vi "GenerateChunks.vi"(9 "Empty Chunk":cluster{cluster{"Last Update":u32, bool}[][][]}, 10 "Point chunk":i32[](array[numeric]), 11 "Map Data in":T1(array[cluster])) -> (3 "Map Data out":T1(array[cluster]))   [LabVIEW 2014]
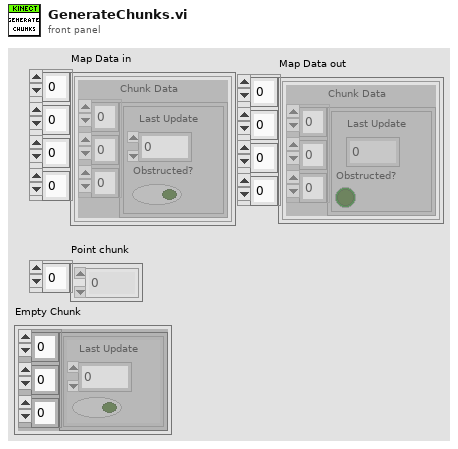
[diagram p1: front panel]
types:
  T1 = cluster{"Chunk Data":cluster{"Last Update":u32, "Obstructed?":bool}[][][]}[][][][]
  T2 = cluster{cluster{"Last Update":u32, bool}[][][]}[][][]
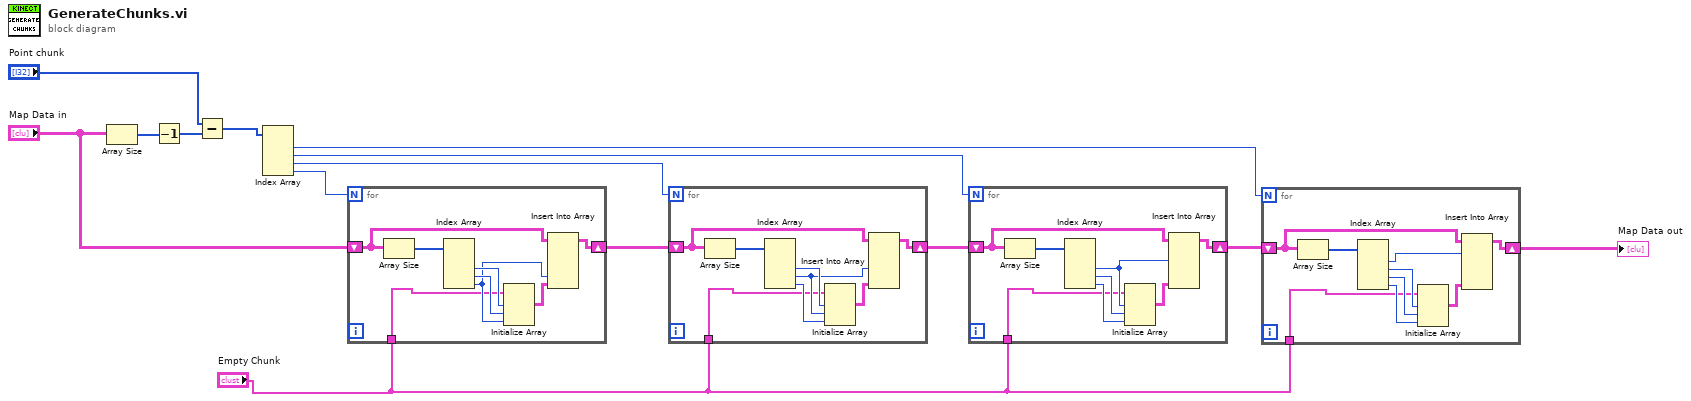
[diagram p0: block diagram]
diagram:
  n1 = Array Size(array="Map Data in") -> (size(s)=w14:i32[])
  n2 = Decrement(x=w14) -> (x-1=w13:i32[])
  n3 = Subtract(x="Point chunk", y=w13) -> (x-y=w4:i32[])
  n4 = Index Array(array=w4) -> (element #1=w11:i32, element #2=w9:i32, element #3=w7:i32, element #4=w6:i32)  [unwired: 4 in]
  n5 = for {
    N: w6 -> [_]
    shift-right: [w22] -> w5
    shift-left: "Map Data in" -> [w19]
    tunnel: "Empty Chunk" -> [w15]
    n6 = Array Size(array=w19) -> (size(s)=w21:i32[])
    n7 = Index Array(array=w21) -> (element #2=w17:i32, element #3=w18:i32, element #4=w16:i32)  [unwired: 4 in, 1 out]
    n8 = Initialize Array(w15, w17, w18, w16) -> (w20:T2)
    n9 = Insert Into Array(array=w19, index (dim 3)=w16, new element=w20) -> (w22:T1)  [unwired: 3 in]
  }
  n10 = for {
    N: w7 -> [_]
    shift-right: [w30] -> w8
    shift-left: w5 -> [w27]
    tunnel: "Empty Chunk" -> [w23]
    n11 = Array Size(array=w27) -> (size(s)=w29:i32[])
    n12 = Index Array(array=w29) -> (element #2=w25:i32, element #3=w24:i32, element #4=w26:i32)  [unwired: 4 in, 1 out]
    n13 = Initialize Array(w23, w25, w24, w26) -> (w28:T2)
    n14 = Insert Into Array(array=w27, index (dim 2)=w24, new element=w28) -> (w30:T1)  [unwired: 3 in]
  }
  n15 = for {
    N: w9 -> [_]
    shift-right: [w38] -> w10
    shift-left: w8 -> [w35]
    tunnel: "Empty Chunk" -> [w31]
    n16 = Array Size(array=w35) -> (size(s)=w37:i32[])
    n17 = Index Array(array=w37) -> (element #2=w32:i32, element #3=w34:i32, element #4=w33:i32)  [unwired: 4 in, 1 out]
    n18 = Initialize Array(w31, w32, w34, w33) -> (w36:T2)
    n19 = Insert Into Array(array=w35, index (dim 1)=w32, new element=w36) -> (w38:T1)  [unwired: 3 in]
  }
  n20 = for {
    N: w11 -> [_]
    shift-right: [w47] -> w1
    shift-left: w10 -> [w44]
    tunnel: "Empty Chunk" -> [w39]
    n21 = Array Size(array=w44) -> (size(s)=w46:i32[])
    n22 = Index Array(array=w46) -> (element #1=w40:i32, element #2=w43:i32, element #3=w42:i32, element #4=w41:i32)  [unwired: 4 in]
    n23 = Initialize Array(w39, w43, w42, w41) -> (w45:T2)
    n24 = Insert Into Array(array=w44, index (dim 0)=w40, new element=w45) -> (w47:T1)  [unwired: 3 in]
  }
  "Map Data out" <- w1
